vi "lab6.vi"() -> ()   [LabVIEW 2020]
panel:
  out "W":dbl(graph)
  out "U":dbl(graph)
  out "I":dbl(graph)
  out "Энергия":dbl
  out "I":dbl(knob) scale=0.0..10.0
  in  "ЭДС":dbl
  in  "L":dbl
  in  "R":dbl
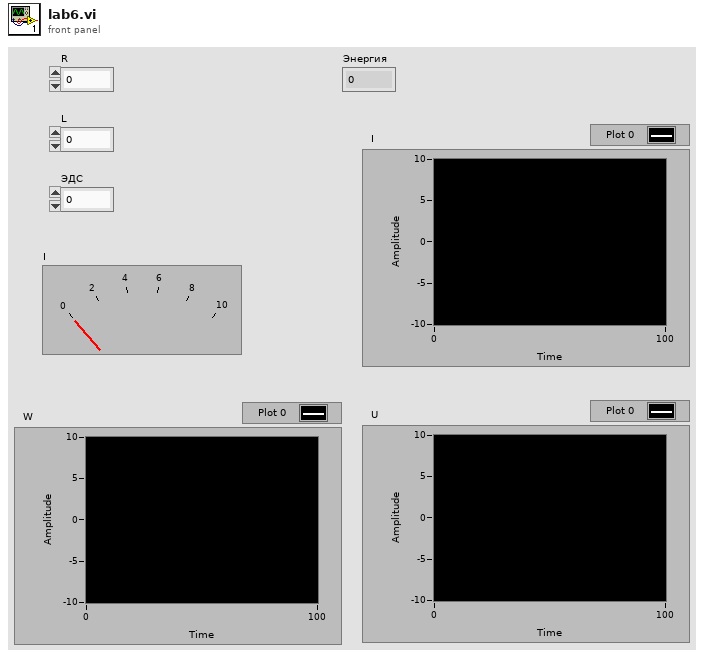
[diagram p1: front panel]
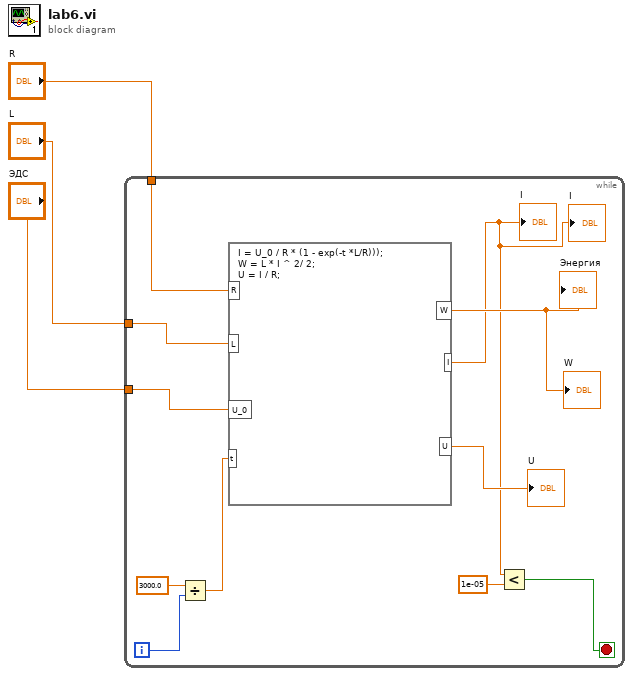
[diagram p0: block diagram]
diagram:
  n1 = while {
    tunnel: "R" -> [w14]
    tunnel: "L" -> [w13]
    tunnel: "ЭДС" -> [w12]
    i -> [w5]
    stop <- w7 stop-if-true
    n2 = Divide(x=3000.0, y=w5) -> (x/y=w4:dbl)
    n3 = formula code="I = U_0 / R * (1 - exp(-t *L/R)));\nW = L * I ^ 2/ 2;\nU = I / R;"("R"=w14, "L"=w13, "U_0"=w12, "t"=w4) -> ("W"=→"Энергия" →"W":dbl, "U"=→"U":dbl, "I"=w9:dbl)
    "I" <- w9
    "I" <- w9
    n4 = Less?(x=w9, y=1e-05) -> (x < y?=w7:bool)
  }
